vi "LED STATUS.vi"() -> ()   [LabVIEW 2023]
uses:
  ctrl defs/ctrl LED STATES.ctl
  <vilib>/Rock Robotics/WPI/DriverStation/WPI_DriverStationRobotMode2.ctl
  Global INIT.vi
  Global stack names.vi
  <vilib>/Rock Robotics/Network Tables/NT Read Boolean.vi
  ctrl defs/ctrl LED PATTERNS.ctl
  <vilib>/Rock Robotics/SystemInterfaces/DIO/FPGA_DIOPWMChannel.ctl
  ctrl defs/ctrl LED init.ctl
panel:
  out "LED init":T1={"PWM Channel"=enum."PWM 0", "refnum name"="LED", "initial output"=0.51, "stack name"="LED/", "Installed?"=FALSE, "pattern"=0} {"pattern" items=["<<Select a pattern>>", "Rainbow, Rainbow palette", "Rainbow, Party palette", "Rainbow, Ocean palette", "Rainbow, Lava palette", "Rainbow, Forest palette", "Rainbow with glitter", "Confetti", "Shot, Red", "Shot, Blue", "Shot, White", "Sinelon, Rainbow palette", "Sinelon, Party palette", "Sinelon, Ocean palette", "Sinelon, Lava palette", "Sinelon, Forest palette", "BPM, Rainbow palette", "BPM, Party palette", "BPM, Ocean palette", "BPM, Lava palette", "BPM, Forest palette", "Fire, Medium", "Fire, Large", "Twinkles, Rainbow palette", "Twinkles, Party palette", "Twinkles, Ocean palette", "Twinkles, Lava palette", "Twinkles, Forest palette", "Color Waves, Rainbow palette", "Color Waves, Party palette", "Color Waves, Ocean palette", "Color Waves, Lava palette", "Color Waves, Forest palette", "Larson Scanner, Red", "Larson Scanner, Gray", "Light Chase, Red", "Light Chase, Blue", "Light Chase, Gray", "Heartbeat, Red", "Heartbeat, Blue", "Heartbeat, White", "Heartbeat, Gray", "Breath, Red", "Breath, Blue", "Breath, Gray", "Strobe, Red", "Strobe, Blue", "Strobe, Gold", "Strobe, White", "Color 1: End to End Blend to Black", "Color 1: Larson Scanner", "Color 1: Light Chase", "Color 1: Heartbeat Slow", "Color 1: Heartbeat Medium", "Color 1: Heartbeat Fast", "Color 1: Breath Slow", "Color 1: Breath Fast", "Color 1: Shot", "Color 1: Strobe", "Color 2: End to End Blend to Black", "Color 2: Larson Scanner", "Color 2: Light Chase", "Color 2: Heartbeat Slow", "Color 2: Heartbeat Medium", "Color 2: Heartbeat Fast", "Color 2: Breath Slow", "Color 2: Breath Fast", "Color 2: Shot", "Color 2: Strobe", "Color 1/2: Sparkle, 1 on 2", "Color 1/2: Sparkle 2 on 1", "Color 1/2: Gradient", "Color 1/2: BPM", "Color 1/2: End to End Blend 1 to 2", "Color 1/2: End to End Blend 2 to 1", "Color 1/2: setup pattern", "Color 1/2: Twinkles", "Color 1/2: Color Waves", "Color 1/2: Sinelon", "Solid Hot Pink", "Solid Dark Red", "Solid Red", "Solid Red Orange", "Solid Orange", "Solid Gold", "Solid Yellow", "Solid Lawn Green", "Solid Lime", "Solid Dark Green", "Solid Green", "Solid Blue Green", "Solid Aqua", "Solid Sky Blue", "Solid Dark Blue", "Solid Blue", "Solid Blue Violet", "Solid Violet", "Solid White", "Solid Gray", "Solid Dark Gray", "Solid Black"]}
  out "LED state":T4
  out "error out":errorcluster
  in  "error in (no error)":errorcluster
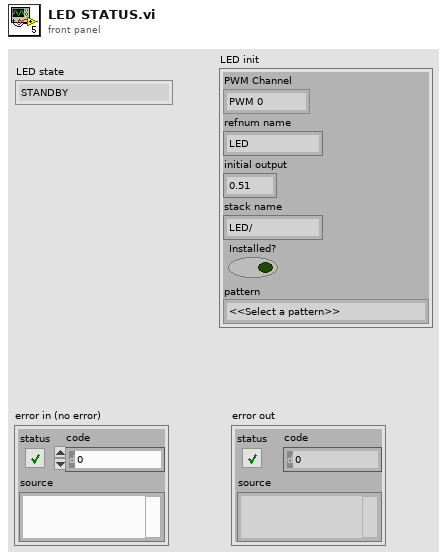
[diagram p1: front panel]
types:
  T1 = typedef "ctrl LED init.ctl" = cluster{"PWM Channel":T2, "refnum name":string, "initial output":dbl, "stack name":string, "Installed?":bool, "pattern":T3}
  T2 = typedef "FPGA_DIOPWMChannel.ctl" = enum8{"PWM 0", "PWM 1", "PWM 2", "PWM 3", "PWM 4", "PWM 5", "PWM 6", "PWM 7", "PWM 8", "PWM 9", "PWM MXP 0", "PWM MXP 1", "PWM MXP 2", "PWM MXP 3", "PWM MXP 4", "PWM MXP 5", "PWM MXP 6", "PWM MXP 7", "PWM MXP 8", "PWM MXP 9", "Invalid"}
  T3 = typedef "ctrl LED PATTERNS.ctl" = u16
  T4 = typedef "ctrl LED STATES.ctl" = enum16{"STANDBY", "END GAME 1", "END GAME 2", "NOTE is LOADED", "LOOKING for NOTE", "PUKE", "EXTENDING ARMS", "RETRACTING ARMS", "ARMS LOCKED", "LOW BATTERY"}
  T5 = typedef "ctrl stack - INTAKE SHOOTER.ctl" = cluster{"INTAKE STATE":string, "RUN INTAKE?":string, "RUN REVERSE?":string, "NOTE LOADED?":string, "SHOOTER STATE":string, "SHOOTER FIRE?":string, "SHOOT AMP?":string, "EXTEND FLAP?":string, "LOOKING for NOTE":string}
  T6 = typedef "WPI_DriverStationRobotMode2.ctl" = enum16{"Autonomous Disabled", "Autonomous Enabled", "Teleop Disabled", "Teleop Enabled", "Disconnected", "Finish", "Test Disabled", "Test Enabled", "Emergency Stopped"}
  T7 = typedef "WPI_DriverStationAllianceInfo.ctl" = enum16{"Red", "Blue", "Invalid"}
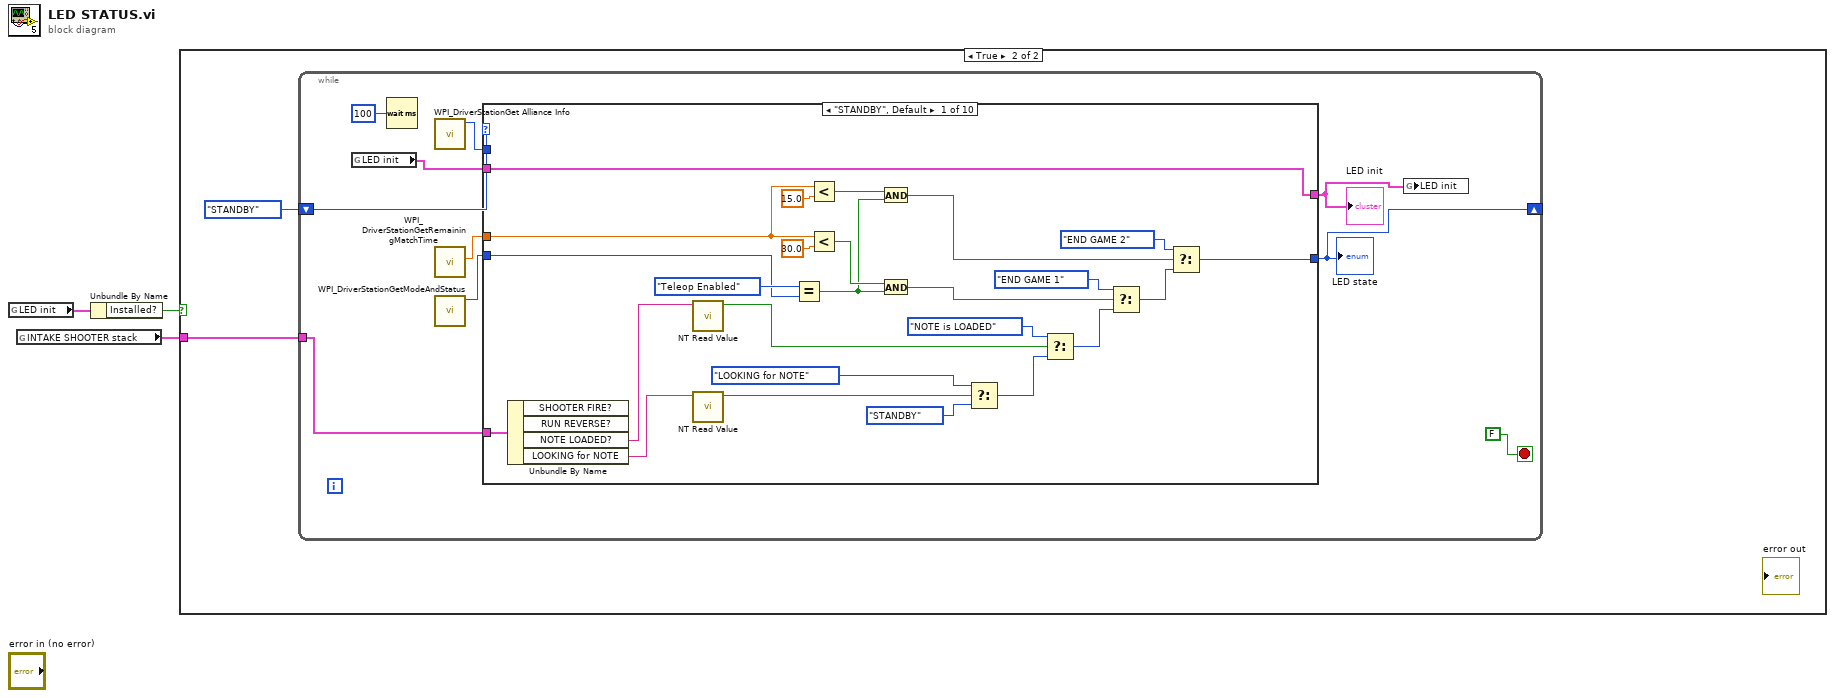
[diagram p0: block diagram]
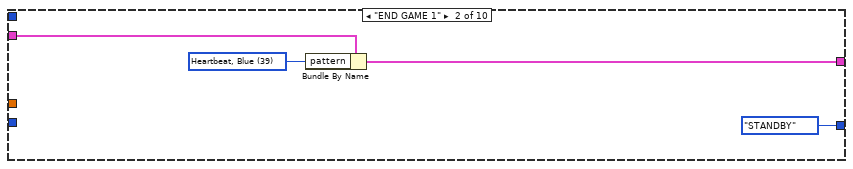
[diagram p3: hidden frame]
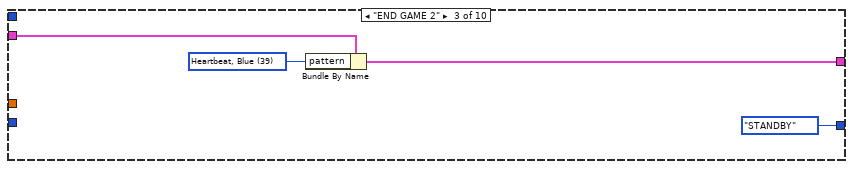
[diagram p4: hidden frame]
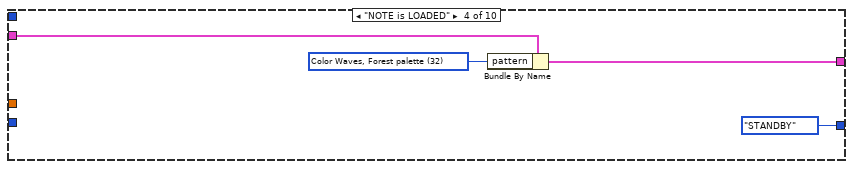
[diagram p5: hidden frame]
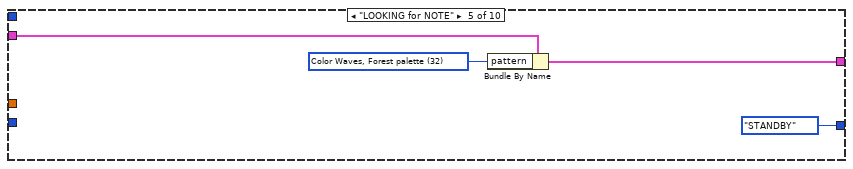
[diagram p6: hidden frame]
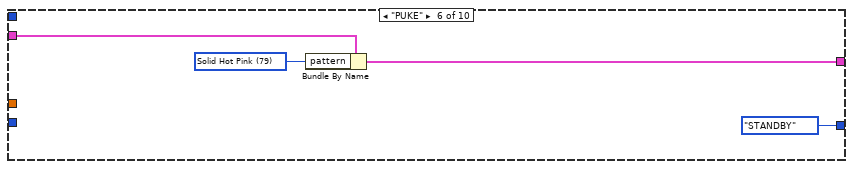
[diagram p7: hidden frame]
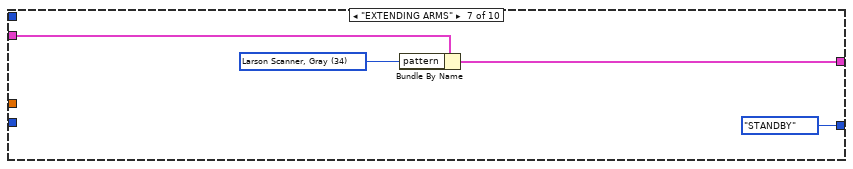
[diagram p8: hidden frame]
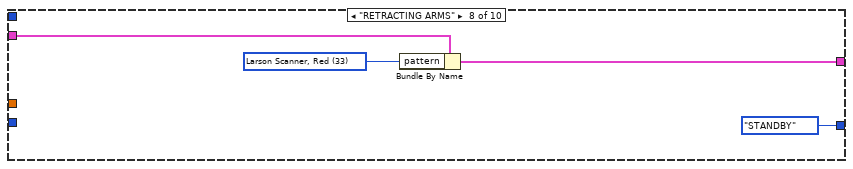
[diagram p9: hidden frame]
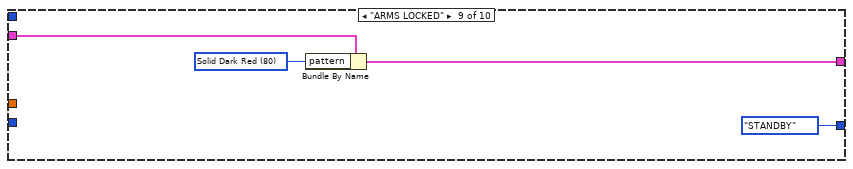
[diagram p10: hidden frame]
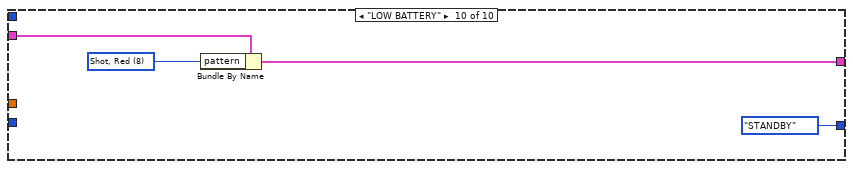
[diagram p11: hidden frame]
diagram:
  n1 = global read "Global INIT.vi" "LED init"() -> (w2:T1)
  n2 = global read "Global stack names.vi" "INTAKE SHOOTER stack"() -> (w1:T5)
  n3 = Unbundle By Name(w2) -> ("Installed?"=w3:bool)
  n4 = case shown="True" w3 {
    tunnel: w1 -> [_ w4]
    frame False {
    }
    frame True {
      n5 = while {
        shift-right: [w9] -> _
        shift-left: ctrl_LED_STATES."STANDBY" -> [w13]
        tunnel: w4 -> [w8]
        stop <- FALSE stop-if-true
        n6 = global read "Global INIT.vi" "LED init"() -> (w7:T1)
        n7 = Wait (ms)(milliseconds to wait=u32 100) -> ()  [unwired: 1 out]
        n8 = call <vilib>:"WPI_DriverStationGet Alliance Info.vi"() -> ("Alliance"=w12:T7)  [unwired: 6 in, 5 out]
        n9 = call <vilib>:"WPI_DriverStationGetRemainingMatchTime.vi"() -> ("Match Time(s)"=w10:sgl)  [unwired: 10 in, 1 out]
        n10 = call <vilib>:"WPI_DriverStationGetModeAndStatus.vi"() -> ("Robot Mode"=w11:T6)  [unwired: 10 in, 1 out]
        n11 = case shown="\"STANDBY\", Default" w13 {
          tunnel: w12 -> [_ _ _ _ _ _ _ _ _ _]
          tunnel: w11 -> [w39 _ _ _ _ _ _ _ _ _]
          tunnel: w10 -> [w34 _ _ _ _ _ _ _ _ _]
          tunnel: [w22 ctrl_LED_STATES."STANDBY" ctrl_LED_STATES."STANDBY" ctrl_LED_STATES."STANDBY" ctrl_LED_STATES."STANDBY" ctrl_LED_STATES."STANDBY" ctrl_LED_STATES."STANDBY" ctrl_LED_STATES."STANDBY" ctrl_LED_STATES."STANDBY" ctrl_LED_STATES."STANDBY"] -> w9
          tunnel: w8 -> [w27 _ _ _ _ _ _ _ _ _]
          tunnel: w7 -> [w21 w42 w45 w51 w54 w57 w61 w65 w69 w73]
          tunnel: [w21 w41 w46 w50 w55 w58 w62 w66 w70 w74] -> w6
          frame "STANDBY", Default {
            n12 = Unbundle By Name(w27) -> ("NOTE LOADED?"=w26:string, "LOOKING for NOTE"=w20:string)  [unwired: 2 out]
            n13 = call-poly <vilib>:"NT Read Value.vi"("name"=w26) -> ("value"=w25:bool)  [unwired: 8 in, 2 out]
            n14 = call-poly <vilib>:"NT Read Value.vi"("name"=w20) -> ("value"=w18:bool)  [unwired: 8 in, 2 out]
            n15 = Equal?(x=WPI_DriverStationRobotMode2."Teleop Enabled" ("Robot Mode"), y=w39) -> (x = y?=w36:bool)
            n16 = Less?(x=w34, y=sgl 15.0) -> (x < y?=w35:bool)
            n17 = Less?(x=w34, y=30.0) -> (x < y?=w37:bool)
            n18 = And(x=w35, y=w36) -> (x .and. y?=w32:bool)
            n19 = And(x=w37, y=w36) -> (x .and. y?=w29:bool)
            n20 = Select(t=ctrl_LED_STATES."LOOKING for NOTE", s=w18, f=ctrl_LED_STATES."STANDBY") -> (s? t:f=w19:T4)
            n21 = Select(t=ctrl_LED_STATES."NOTE is LOADED", s=w25, f=w19) -> (s? t:f=w23:T4)
            n22 = Select(t=ctrl_LED_STATES."END GAME 1", s=w29, f=w23) -> (s? t:f=w30:T4)
            n23 = Select(t=ctrl_LED_STATES."END GAME 2", s=w32, f=w30) -> (s? t:f=w22:T4)
          }
          frame "END GAME 1" {
            w43 = T3 39 items=["<<Select a pattern>>", "Rainbow, Rainbow palette", "Rainbow, Party palette", "Rainbow, Ocean palette", "Rainbow, Lava palette", "Rainbow, Forest palette", "Rainbow with glitter", "Confetti", "Shot, Red", "Shot, Blue", "Shot, White", "Sinelon, Rainbow palette", "Sinelon, Party palette", "Sinelon, Ocean palette", "Sinelon, Lava palette", "Sinelon, Forest palette", "BPM, Rainbow palette", "BPM, Party palette", "BPM, Ocean palette", "BPM, Lava palette", "BPM, Forest palette", "Fire, Medium", "Fire, Large", "Twinkles, Rainbow palette", "Twinkles, Party palette", "Twinkles, Ocean palette", "Twinkles, Lava palette", "Twinkles, Forest palette", "Color Waves, Rainbow palette", "Color Waves, Party palette", "Color Waves, Ocean palette", "Color Waves, Lava palette", "Color Waves, Forest palette", "Larson Scanner, Red", "Larson Scanner, Gray", "Light Chase, Red", "Light Chase, Blue", "Light Chase, Gray", "Heartbeat, Red", "Heartbeat, Blue", "Heartbeat, White", "Heartbeat, Gray", "Breath, Red", "Breath, Blue", "Breath, Gray", "Strobe, Red", "Strobe, Blue", "Strobe, Gold", "Strobe, White", "Color 1: End to End Blend to Black", "Color 1: Larson Scanner", "Color 1: Light Chase", "Color 1: Heartbeat Slow", "Color 1: Heartbeat Medium", "Color 1: Heartbeat Fast", "Color 1: Breath Slow", "Color 1: Breath Fast", "Color 1: Shot", "Color 1: Strobe", "Color 2: End to End Blend to Black", "Color 2: Larson Scanner", "Color 2: Light Chase", "Color 2: Heartbeat Slow", "Color 2: Heartbeat Medium", "Color 2: Heartbeat Fast", "Color 2: Breath Slow", "Color 2: Breath Fast", "Color 2: Shot", "Color 2: Strobe", "Color 1/2: Sparkle, 1 on 2", "Color 1/2: Sparkle 2 on 1", "Color 1/2: Gradient", "Color 1/2: BPM", "Color 1/2: End to End Blend 1 to 2", "Color 1/2: End to End Blend 2 to 1", "Color 1/2: setup pattern", "Color 1/2: Twinkles", "Color 1/2: Color Waves", "Color 1/2: Sinelon", "Solid Hot Pink", "Solid Dark Red", "Solid Red", "Solid Red Orange", "Solid Orange", "Solid Gold", "Solid Yellow", "Solid Lawn Green", "Solid Lime", "Solid Dark Green", "Solid Green", "Solid Blue Green", "Solid Aqua", "Solid Sky Blue", "Solid Dark Blue", "Solid Blue", "Solid Blue Violet", "Solid Violet", "Solid White", "Solid Gray", "Solid Dark Gray", "Solid Black"] ("pattern")
            n24 = Bundle By Name(cluster=w42, "pattern"=w43) -> (w41:T1)
          }
          frame "END GAME 2" {
            w47 = T3 39 items=["<<Select a pattern>>", "Rainbow, Rainbow palette", "Rainbow, Party palette", "Rainbow, Ocean palette", "Rainbow, Lava palette", "Rainbow, Forest palette", "Rainbow with glitter", "Confetti", "Shot, Red", "Shot, Blue", "Shot, White", "Sinelon, Rainbow palette", "Sinelon, Party palette", "Sinelon, Ocean palette", "Sinelon, Lava palette", "Sinelon, Forest palette", "BPM, Rainbow palette", "BPM, Party palette", "BPM, Ocean palette", "BPM, Lava palette", "BPM, Forest palette", "Fire, Medium", "Fire, Large", "Twinkles, Rainbow palette", "Twinkles, Party palette", "Twinkles, Ocean palette", "Twinkles, Lava palette", "Twinkles, Forest palette", "Color Waves, Rainbow palette", "Color Waves, Party palette", "Color Waves, Ocean palette", "Color Waves, Lava palette", "Color Waves, Forest palette", "Larson Scanner, Red", "Larson Scanner, Gray", "Light Chase, Red", "Light Chase, Blue", "Light Chase, Gray", "Heartbeat, Red", "Heartbeat, Blue", "Heartbeat, White", "Heartbeat, Gray", "Breath, Red", "Breath, Blue", "Breath, Gray", "Strobe, Red", "Strobe, Blue", "Strobe, Gold", "Strobe, White", "Color 1: End to End Blend to Black", "Color 1: Larson Scanner", "Color 1: Light Chase", "Color 1: Heartbeat Slow", "Color 1: Heartbeat Medium", "Color 1: Heartbeat Fast", "Color 1: Breath Slow", "Color 1: Breath Fast", "Color 1: Shot", "Color 1: Strobe", "Color 2: End to End Blend to Black", "Color 2: Larson Scanner", "Color 2: Light Chase", "Color 2: Heartbeat Slow", "Color 2: Heartbeat Medium", "Color 2: Heartbeat Fast", "Color 2: Breath Slow", "Color 2: Breath Fast", "Color 2: Shot", "Color 2: Strobe", "Color 1/2: Sparkle, 1 on 2", "Color 1/2: Sparkle 2 on 1", "Color 1/2: Gradient", "Color 1/2: BPM", "Color 1/2: End to End Blend 1 to 2", "Color 1/2: End to End Blend 2 to 1", "Color 1/2: setup pattern", "Color 1/2: Twinkles", "Color 1/2: Color Waves", "Color 1/2: Sinelon", "Solid Hot Pink", "Solid Dark Red", "Solid Red", "Solid Red Orange", "Solid Orange", "Solid Gold", "Solid Yellow", "Solid Lawn Green", "Solid Lime", "Solid Dark Green", "Solid Green", "Solid Blue Green", "Solid Aqua", "Solid Sky Blue", "Solid Dark Blue", "Solid Blue", "Solid Blue Violet", "Solid Violet", "Solid White", "Solid Gray", "Solid Dark Gray", "Solid Black"] ("pattern")
            n25 = Bundle By Name(cluster=w45, "pattern"=w47) -> (w46:T1)
          }
          frame "NOTE is LOADED" {
            w49 = T3 32 items=["<<Select a pattern>>", "Rainbow, Rainbow palette", "Rainbow, Party palette", "Rainbow, Ocean palette", "Rainbow, Lava palette", "Rainbow, Forest palette", "Rainbow with glitter", "Confetti", "Shot, Red", "Shot, Blue", "Shot, White", "Sinelon, Rainbow palette", "Sinelon, Party palette", "Sinelon, Ocean palette", "Sinelon, Lava palette", "Sinelon, Forest palette", "BPM, Rainbow palette", "BPM, Party palette", "BPM, Ocean palette", "BPM, Lava palette", "BPM, Forest palette", "Fire, Medium", "Fire, Large", "Twinkles, Rainbow palette", "Twinkles, Party palette", "Twinkles, Ocean palette", "Twinkles, Lava palette", "Twinkles, Forest palette", "Color Waves, Rainbow palette", "Color Waves, Party palette", "Color Waves, Ocean palette", "Color Waves, Lava palette", "Color Waves, Forest palette", "Larson Scanner, Red", "Larson Scanner, Gray", "Light Chase, Red", "Light Chase, Blue", "Light Chase, Gray", "Heartbeat, Red", "Heartbeat, Blue", "Heartbeat, White", "Heartbeat, Gray", "Breath, Red", "Breath, Blue", "Breath, Gray", "Strobe, Red", "Strobe, Blue", "Strobe, Gold", "Strobe, White", "Color 1: End to End Blend to Black", "Color 1: Larson Scanner", "Color 1: Light Chase", "Color 1: Heartbeat Slow", "Color 1: Heartbeat Medium", "Color 1: Heartbeat Fast", "Color 1: Breath Slow", "Color 1: Breath Fast", "Color 1: Shot", "Color 1: Strobe", "Color 2: End to End Blend to Black", "Color 2: Larson Scanner", "Color 2: Light Chase", "Color 2: Heartbeat Slow", "Color 2: Heartbeat Medium", "Color 2: Heartbeat Fast", "Color 2: Breath Slow", "Color 2: Breath Fast", "Color 2: Shot", "Color 2: Strobe", "Color 1/2: Sparkle, 1 on 2", "Color 1/2: Sparkle 2 on 1", "Color 1/2: Gradient", "Color 1/2: BPM", "Color 1/2: End to End Blend 1 to 2", "Color 1/2: End to End Blend 2 to 1", "Color 1/2: setup pattern", "Color 1/2: Twinkles", "Color 1/2: Color Waves", "Color 1/2: Sinelon", "Solid Hot Pink", "Solid Dark Red", "Solid Red", "Solid Red Orange", "Solid Orange", "Solid Gold", "Solid Yellow", "Solid Lawn Green", "Solid Lime", "Solid Dark Green", "Solid Green", "Solid Blue Green", "Solid Aqua", "Solid Sky Blue", "Solid Dark Blue", "Solid Blue", "Solid Blue Violet", "Solid Violet", "Solid White", "Solid Gray", "Solid Dark Gray", "Solid Black"] ("pattern")
            n26 = Bundle By Name(cluster=w51, "pattern"=w49) -> (w50:T1)
          }
          frame "LOOKING for NOTE" {
            w56 = T3 32 items=["<<Select a pattern>>", "Rainbow, Rainbow palette", "Rainbow, Party palette", "Rainbow, Ocean palette", "Rainbow, Lava palette", "Rainbow, Forest palette", "Rainbow with glitter", "Confetti", "Shot, Red", "Shot, Blue", "Shot, White", "Sinelon, Rainbow palette", "Sinelon, Party palette", "Sinelon, Ocean palette", "Sinelon, Lava palette", "Sinelon, Forest palette", "BPM, Rainbow palette", "BPM, Party palette", "BPM, Ocean palette", "BPM, Lava palette", "BPM, Forest palette", "Fire, Medium", "Fire, Large", "Twinkles, Rainbow palette", "Twinkles, Party palette", "Twinkles, Ocean palette", "Twinkles, Lava palette", "Twinkles, Forest palette", "Color Waves, Rainbow palette", "Color Waves, Party palette", "Color Waves, Ocean palette", "Color Waves, Lava palette", "Color Waves, Forest palette", "Larson Scanner, Red", "Larson Scanner, Gray", "Light Chase, Red", "Light Chase, Blue", "Light Chase, Gray", "Heartbeat, Red", "Heartbeat, Blue", "Heartbeat, White", "Heartbeat, Gray", "Breath, Red", "Breath, Blue", "Breath, Gray", "Strobe, Red", "Strobe, Blue", "Strobe, Gold", "Strobe, White", "Color 1: End to End Blend to Black", "Color 1: Larson Scanner", "Color 1: Light Chase", "Color 1: Heartbeat Slow", "Color 1: Heartbeat Medium", "Color 1: Heartbeat Fast", "Color 1: Breath Slow", "Color 1: Breath Fast", "Color 1: Shot", "Color 1: Strobe", "Color 2: End to End Blend to Black", "Color 2: Larson Scanner", "Color 2: Light Chase", "Color 2: Heartbeat Slow", "Color 2: Heartbeat Medium", "Color 2: Heartbeat Fast", "Color 2: Breath Slow", "Color 2: Breath Fast", "Color 2: Shot", "Color 2: Strobe", "Color 1/2: Sparkle, 1 on 2", "Color 1/2: Sparkle 2 on 1", "Color 1/2: Gradient", "Color 1/2: BPM", "Color 1/2: End to End Blend 1 to 2", "Color 1/2: End to End Blend 2 to 1", "Color 1/2: setup pattern", "Color 1/2: Twinkles", "Color 1/2: Color Waves", "Color 1/2: Sinelon", "Solid Hot Pink", "Solid Dark Red", "Solid Red", "Solid Red Orange", "Solid Orange", "Solid Gold", "Solid Yellow", "Solid Lawn Green", "Solid Lime", "Solid Dark Green", "Solid Green", "Solid Blue Green", "Solid Aqua", "Solid Sky Blue", "Solid Dark Blue", "Solid Blue", "Solid Blue Violet", "Solid Violet", "Solid White", "Solid Gray", "Solid Dark Gray", "Solid Black"] ("pattern")
            n27 = Bundle By Name(cluster=w54, "pattern"=w56) -> (w55:T1)
          }
          frame "PUKE" {
            w59 = T3 79 items=["<<Select a pattern>>", "Rainbow, Rainbow palette", "Rainbow, Party palette", "Rainbow, Ocean palette", "Rainbow, Lava palette", "Rainbow, Forest palette", "Rainbow with glitter", "Confetti", "Shot, Red", "Shot, Blue", "Shot, White", "Sinelon, Rainbow palette", "Sinelon, Party palette", "Sinelon, Ocean palette", "Sinelon, Lava palette", "Sinelon, Forest palette", "BPM, Rainbow palette", "BPM, Party palette", "BPM, Ocean palette", "BPM, Lava palette", "BPM, Forest palette", "Fire, Medium", "Fire, Large", "Twinkles, Rainbow palette", "Twinkles, Party palette", "Twinkles, Ocean palette", "Twinkles, Lava palette", "Twinkles, Forest palette", "Color Waves, Rainbow palette", "Color Waves, Party palette", "Color Waves, Ocean palette", "Color Waves, Lava palette", "Color Waves, Forest palette", "Larson Scanner, Red", "Larson Scanner, Gray", "Light Chase, Red", "Light Chase, Blue", "Light Chase, Gray", "Heartbeat, Red", "Heartbeat, Blue", "Heartbeat, White", "Heartbeat, Gray", "Breath, Red", "Breath, Blue", "Breath, Gray", "Strobe, Red", "Strobe, Blue", "Strobe, Gold", "Strobe, White", "Color 1: End to End Blend to Black", "Color 1: Larson Scanner", "Color 1: Light Chase", "Color 1: Heartbeat Slow", "Color 1: Heartbeat Medium", "Color 1: Heartbeat Fast", "Color 1: Breath Slow", "Color 1: Breath Fast", "Color 1: Shot", "Color 1: Strobe", "Color 2: End to End Blend to Black", "Color 2: Larson Scanner", "Color 2: Light Chase", "Color 2: Heartbeat Slow", "Color 2: Heartbeat Medium", "Color 2: Heartbeat Fast", "Color 2: Breath Slow", "Color 2: Breath Fast", "Color 2: Shot", "Color 2: Strobe", "Color 1/2: Sparkle, 1 on 2", "Color 1/2: Sparkle 2 on 1", "Color 1/2: Gradient", "Color 1/2: BPM", "Color 1/2: End to End Blend 1 to 2", "Color 1/2: End to End Blend 2 to 1", "Color 1/2: setup pattern", "Color 1/2: Twinkles", "Color 1/2: Color Waves", "Color 1/2: Sinelon", "Solid Hot Pink", "Solid Dark Red", "Solid Red", "Solid Red Orange", "Solid Orange", "Solid Gold", "Solid Yellow", "Solid Lawn Green", "Solid Lime", "Solid Dark Green", "Solid Green", "Solid Blue Green", "Solid Aqua", "Solid Sky Blue", "Solid Dark Blue", "Solid Blue", "Solid Blue Violet", "Solid Violet", "Solid White", "Solid Gray", "Solid Dark Gray", "Solid Black"] ("pattern")
            n28 = Bundle By Name(cluster=w57, "pattern"=w59) -> (w58:T1)
          }
          frame "EXTENDING ARMS" {
            w64 = T3 34 items=["<<Select a pattern>>", "Rainbow, Rainbow palette", "Rainbow, Party palette", "Rainbow, Ocean palette", "Rainbow, Lava palette", "Rainbow, Forest palette", "Rainbow with glitter", "Confetti", "Shot, Red", "Shot, Blue", "Shot, White", "Sinelon, Rainbow palette", "Sinelon, Party palette", "Sinelon, Ocean palette", "Sinelon, Lava palette", "Sinelon, Forest palette", "BPM, Rainbow palette", "BPM, Party palette", "BPM, Ocean palette", "BPM, Lava palette", "BPM, Forest palette", "Fire, Medium", "Fire, Large", "Twinkles, Rainbow palette", "Twinkles, Party palette", "Twinkles, Ocean palette", "Twinkles, Lava palette", "Twinkles, Forest palette", "Color Waves, Rainbow palette", "Color Waves, Party palette", "Color Waves, Ocean palette", "Color Waves, Lava palette", "Color Waves, Forest palette", "Larson Scanner, Red", "Larson Scanner, Gray", "Light Chase, Red", "Light Chase, Blue", "Light Chase, Gray", "Heartbeat, Red", "Heartbeat, Blue", "Heartbeat, White", "Heartbeat, Gray", "Breath, Red", "Breath, Blue", "Breath, Gray", "Strobe, Red", "Strobe, Blue", "Strobe, Gold", "Strobe, White", "Color 1: End to End Blend to Black", "Color 1: Larson Scanner", "Color 1: Light Chase", "Color 1: Heartbeat Slow", "Color 1: Heartbeat Medium", "Color 1: Heartbeat Fast", "Color 1: Breath Slow", "Color 1: Breath Fast", "Color 1: Shot", "Color 1: Strobe", "Color 2: End to End Blend to Black", "Color 2: Larson Scanner", "Color 2: Light Chase", "Color 2: Heartbeat Slow", "Color 2: Heartbeat Medium", "Color 2: Heartbeat Fast", "Color 2: Breath Slow", "Color 2: Breath Fast", "Color 2: Shot", "Color 2: Strobe", "Color 1/2: Sparkle, 1 on 2", "Color 1/2: Sparkle 2 on 1", "Color 1/2: Gradient", "Color 1/2: BPM", "Color 1/2: End to End Blend 1 to 2", "Color 1/2: End to End Blend 2 to 1", "Color 1/2: setup pattern", "Color 1/2: Twinkles", "Color 1/2: Color Waves", "Color 1/2: Sinelon", "Solid Hot Pink", "Solid Dark Red", "Solid Red", "Solid Red Orange", "Solid Orange", "Solid Gold", "Solid Yellow", "Solid Lawn Green", "Solid Lime", "Solid Dark Green", "Solid Green", "Solid Blue Green", "Solid Aqua", "Solid Sky Blue", "Solid Dark Blue", "Solid Blue", "Solid Blue Violet", "Solid Violet", "Solid White", "Solid Gray", "Solid Dark Gray", "Solid Black"] ("pattern")
            n29 = Bundle By Name(cluster=w61, "pattern"=w64) -> (w62:T1)
          }
          frame "RETRACTING ARMS" {
            w67 = T3 33 items=["<<Select a pattern>>", "Rainbow, Rainbow palette", "Rainbow, Party palette", "Rainbow, Ocean palette", "Rainbow, Lava palette", "Rainbow, Forest palette", "Rainbow with glitter", "Confetti", "Shot, Red", "Shot, Blue", "Shot, White", "Sinelon, Rainbow palette", "Sinelon, Party palette", "Sinelon, Ocean palette", "Sinelon, Lava palette", "Sinelon, Forest palette", "BPM, Rainbow palette", "BPM, Party palette", "BPM, Ocean palette", "BPM, Lava palette", "BPM, Forest palette", "Fire, Medium", "Fire, Large", "Twinkles, Rainbow palette", "Twinkles, Party palette", "Twinkles, Ocean palette", "Twinkles, Lava palette", "Twinkles, Forest palette", "Color Waves, Rainbow palette", "Color Waves, Party palette", "Color Waves, Ocean palette", "Color Waves, Lava palette", "Color Waves, Forest palette", "Larson Scanner, Red", "Larson Scanner, Gray", "Light Chase, Red", "Light Chase, Blue", "Light Chase, Gray", "Heartbeat, Red", "Heartbeat, Blue", "Heartbeat, White", "Heartbeat, Gray", "Breath, Red", "Breath, Blue", "Breath, Gray", "Strobe, Red", "Strobe, Blue", "Strobe, Gold", "Strobe, White", "Color 1: End to End Blend to Black", "Color 1: Larson Scanner", "Color 1: Light Chase", "Color 1: Heartbeat Slow", "Color 1: Heartbeat Medium", "Color 1: Heartbeat Fast", "Color 1: Breath Slow", "Color 1: Breath Fast", "Color 1: Shot", "Color 1: Strobe", "Color 2: End to End Blend to Black", "Color 2: Larson Scanner", "Color 2: Light Chase", "Color 2: Heartbeat Slow", "Color 2: Heartbeat Medium", "Color 2: Heartbeat Fast", "Color 2: Breath Slow", "Color 2: Breath Fast", "Color 2: Shot", "Color 2: Strobe", "Color 1/2: Sparkle, 1 on 2", "Color 1/2: Sparkle 2 on 1", "Color 1/2: Gradient", "Color 1/2: BPM", "Color 1/2: End to End Blend 1 to 2", "Color 1/2: End to End Blend 2 to 1", "Color 1/2: setup pattern", "Color 1/2: Twinkles", "Color 1/2: Color Waves", "Color 1/2: Sinelon", "Solid Hot Pink", "Solid Dark Red", "Solid Red", "Solid Red Orange", "Solid Orange", "Solid Gold", "Solid Yellow", "Solid Lawn Green", "Solid Lime", "Solid Dark Green", "Solid Green", "Solid Blue Green", "Solid Aqua", "Solid Sky Blue", "Solid Dark Blue", "Solid Blue", "Solid Blue Violet", "Solid Violet", "Solid White", "Solid Gray", "Solid Dark Gray", "Solid Black"] ("pattern")
            n30 = Bundle By Name(cluster=w65, "pattern"=w67) -> (w66:T1)
          }
          frame "ARMS LOCKED" {
            w71 = T3 80 items=["<<Select a pattern>>", "Rainbow, Rainbow palette", "Rainbow, Party palette", "Rainbow, Ocean palette", "Rainbow, Lava palette", "Rainbow, Forest palette", "Rainbow with glitter", "Confetti", "Shot, Red", "Shot, Blue", "Shot, White", "Sinelon, Rainbow palette", "Sinelon, Party palette", "Sinelon, Ocean palette", "Sinelon, Lava palette", "Sinelon, Forest palette", "BPM, Rainbow palette", "BPM, Party palette", "BPM, Ocean palette", "BPM, Lava palette", "BPM, Forest palette", "Fire, Medium", "Fire, Large", "Twinkles, Rainbow palette", "Twinkles, Party palette", "Twinkles, Ocean palette", "Twinkles, Lava palette", "Twinkles, Forest palette", "Color Waves, Rainbow palette", "Color Waves, Party palette", "Color Waves, Ocean palette", "Color Waves, Lava palette", "Color Waves, Forest palette", "Larson Scanner, Red", "Larson Scanner, Gray", "Light Chase, Red", "Light Chase, Blue", "Light Chase, Gray", "Heartbeat, Red", "Heartbeat, Blue", "Heartbeat, White", "Heartbeat, Gray", "Breath, Red", "Breath, Blue", "Breath, Gray", "Strobe, Red", "Strobe, Blue", "Strobe, Gold", "Strobe, White", "Color 1: End to End Blend to Black", "Color 1: Larson Scanner", "Color 1: Light Chase", "Color 1: Heartbeat Slow", "Color 1: Heartbeat Medium", "Color 1: Heartbeat Fast", "Color 1: Breath Slow", "Color 1: Breath Fast", "Color 1: Shot", "Color 1: Strobe", "Color 2: End to End Blend to Black", "Color 2: Larson Scanner", "Color 2: Light Chase", "Color 2: Heartbeat Slow", "Color 2: Heartbeat Medium", "Color 2: Heartbeat Fast", "Color 2: Breath Slow", "Color 2: Breath Fast", "Color 2: Shot", "Color 2: Strobe", "Color 1/2: Sparkle, 1 on 2", "Color 1/2: Sparkle 2 on 1", "Color 1/2: Gradient", "Color 1/2: BPM", "Color 1/2: End to End Blend 1 to 2", "Color 1/2: End to End Blend 2 to 1", "Color 1/2: setup pattern", "Color 1/2: Twinkles", "Color 1/2: Color Waves", "Color 1/2: Sinelon", "Solid Hot Pink", "Solid Dark Red", "Solid Red", "Solid Red Orange", "Solid Orange", "Solid Gold", "Solid Yellow", "Solid Lawn Green", "Solid Lime", "Solid Dark Green", "Solid Green", "Solid Blue Green", "Solid Aqua", "Solid Sky Blue", "Solid Dark Blue", "Solid Blue", "Solid Blue Violet", "Solid Violet", "Solid White", "Solid Gray", "Solid Dark Gray", "Solid Black"] ("pattern")
            n31 = Bundle By Name(cluster=w69, "pattern"=w71) -> (w70:T1)
          }
          frame "LOW BATTERY" {
            w75 = T3 8 items=["<<Select a pattern>>", "Rainbow, Rainbow palette", "Rainbow, Party palette", "Rainbow, Ocean palette", "Rainbow, Lava palette", "Rainbow, Forest palette", "Rainbow with glitter", "Confetti", "Shot, Red", "Shot, Blue", "Shot, White", "Sinelon, Rainbow palette", "Sinelon, Party palette", "Sinelon, Ocean palette", "Sinelon, Lava palette", "Sinelon, Forest palette", "BPM, Rainbow palette", "BPM, Party palette", "BPM, Ocean palette", "BPM, Lava palette", "BPM, Forest palette", "Fire, Medium", "Fire, Large", "Twinkles, Rainbow palette", "Twinkles, Party palette", "Twinkles, Ocean palette", "Twinkles, Lava palette", "Twinkles, Forest palette", "Color Waves, Rainbow palette", "Color Waves, Party palette", "Color Waves, Ocean palette", "Color Waves, Lava palette", "Color Waves, Forest palette", "Larson Scanner, Red", "Larson Scanner, Gray", "Light Chase, Red", "Light Chase, Blue", "Light Chase, Gray", "Heartbeat, Red", "Heartbeat, Blue", "Heartbeat, White", "Heartbeat, Gray", "Breath, Red", "Breath, Blue", "Breath, Gray", "Strobe, Red", "Strobe, Blue", "Strobe, Gold", "Strobe, White", "Color 1: End to End Blend to Black", "Color 1: Larson Scanner", "Color 1: Light Chase", "Color 1: Heartbeat Slow", "Color 1: Heartbeat Medium", "Color 1: Heartbeat Fast", "Color 1: Breath Slow", "Color 1: Breath Fast", "Color 1: Shot", "Color 1: Strobe", "Color 2: End to End Blend to Black", "Color 2: Larson Scanner", "Color 2: Light Chase", "Color 2: Heartbeat Slow", "Color 2: Heartbeat Medium", "Color 2: Heartbeat Fast", "Color 2: Breath Slow", "Color 2: Breath Fast", "Color 2: Shot", "Color 2: Strobe", "Color 1/2: Sparkle, 1 on 2", "Color 1/2: Sparkle 2 on 1", "Color 1/2: Gradient", "Color 1/2: BPM", "Color 1/2: End to End Blend 1 to 2", "Color 1/2: End to End Blend 2 to 1", "Color 1/2: setup pattern", "Color 1/2: Twinkles", "Color 1/2: Color Waves", "Color 1/2: Sinelon", "Solid Hot Pink", "Solid Dark Red", "Solid Red", "Solid Red Orange", "Solid Orange", "Solid Gold", "Solid Yellow", "Solid Lawn Green", "Solid Lime", "Solid Dark Green", "Solid Green", "Solid Blue Green", "Solid Aqua", "Solid Sky Blue", "Solid Dark Blue", "Solid Blue", "Solid Blue Violet", "Solid Violet", "Solid White", "Solid Gray", "Solid Dark Gray", "Solid Black"] ("pattern")
            n32 = Bundle By Name(cluster=w73, "pattern"=w75) -> (w74:T1)
          }
        }
        "LED state" <- w9
        "LED init" <- w6
        n33 = global write "Global INIT.vi" "LED init"(w6) -> ()
      }
    }
  }
